vi "DSF.Engine.Framework.Create.Plugins.vi"(8 "error in (no error)":errorcluster, 10 "Plugin Configurations":refnum<class "DSF.Shared.Configuration.Plugin.lvclass">[](array[class]), 11 "Framework in":refnum<class "DSF.Engine.Framework.lvclass">) -> (0 "error out":errorcluster, 2 "Plugins":refnum<class "DSF.Engine.Plugin.lvclass">[](array[class]), 3 "Framework out":refnum<class "DSF.Engine.Framework.lvclass">)   [LabVIEW 2017, in "DSF.Engine.lvlib" / "DSF.Engine.Framework.lvclass"]
uses:
  DSF.Engine.Framework.lvclass
  Shared/Classes/Plugin/DSF.Shared.Configuration.Plugin.lvclass
  Plugin/DSF.Engine.Plugin.lvclass
  Plugins/UDP/DSF.Transceiver.UDP.lvclass
  C:/Git/DSF/Source/Engine/Classes/Transceiver/DSF.Engine.Transceiver.lvclass
  Shared/Classes/Plugin/DSF.Shared.Configuration.Plugin.lvclass/DSF.Shared.Configuration.Plugin.ctl
  DSF.Engine.Framework.lvclass/DSF.Engine.Framework.ctl
  Timing/DSF.Engine.Timing.lvclass
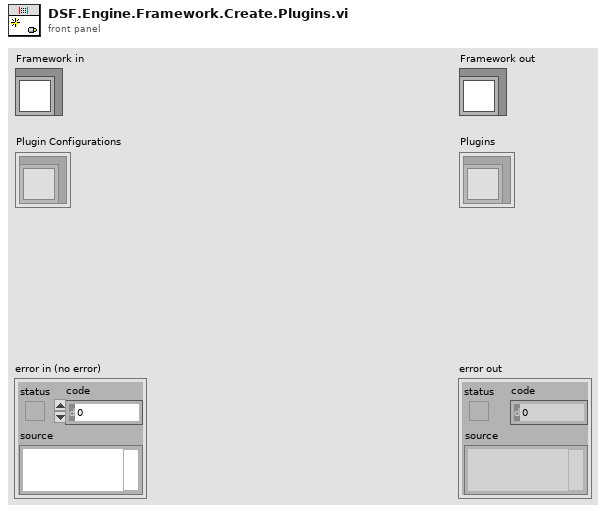
[diagram p1: front panel]
types:
  T1 = typedef "DSF.Shared.lvlib/DSF.Shared.Typedefs.Cycle Timing Factors.ctl" = cluster{"Priority":u64, "Decimation":u64, "Offset":u64}
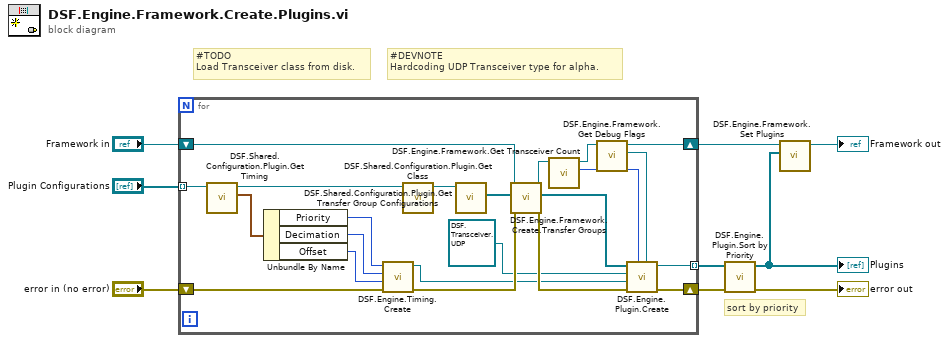
[diagram p0: block diagram]
diagram:
  # "#TODO\nLoad Transceiver class from disk."
  # "#DEVNOTE\nHardcoding UDP Transceiver type for alpha."
  # "sort by priority"
  n1 = for {
    shift-right: [w25] -> w7
    shift-left: "error in (no error)" -> [w26]
    shift-right: [w12] -> w3
    shift-left: "Framework in" -> [w21]
    tunnel: "Plugin Configurations" -> [w31] mode=indexing
    tunnel: [w17] -> w2 mode=indexing
    n2 = call "DSF.Shared.Configuration.Plugin.Get Timing.vi"("Plugin Configuration in"=w31) -> ("cycle timing"=w30:T1, "Plugin Configuration out"=w24:refnum<class "DSF.Shared.Configuration.Plugin.lvclass">)  [unwired: 9 in]
    n3 = Unbundle By Name(w30) -> ("Priority"=w27:u64, "Decimation"=w28:u64, "Offset"=w29:u64)
    n4 = call "DSF.Engine.Timing.Create.vi"("error in (no error)"=w26, "Offset"=w29, "Decimation"=w28, "Priority"=w27) -> ("error out"=w19:errorcluster, "Timing"=w16:refnum<class "DSF.Engine.Timing.lvclass">)  [unwired: 6 in]
    n5 = call "DSF.Shared.Configuration.Plugin.Get Class.vi"("Plugin Configuration in"=w24) -> ("Plugin Configuration out"=w23:refnum<class "DSF.Shared.Configuration.Plugin.lvclass">)  [unwired: 9 in, 1 out]
    n6 = call "DSF.Shared.Configuration.Plugin.Get Transfer Group Configurations.vi"("Plugin Configuration in"=w23) -> ("Transfer Group Configurations"=w22:refnum<class "DSF.Shared.Configuration.Transfer Group.lvclass">[])  [unwired: 9 in, 1 out]
    n7 = call "DSF.Engine.Framework.Create.Transfer Groups.vi"("error in (no error)"=w19, "Transfer Group Configurations"=w22, "Framework in"=w21) -> ("error out"=w18:errorcluster, "Transfer Groups"=w20:refnum<class "DSF.Engine.Transfer Group.lvclass">[], "Framework out"=w14:refnum<class "DSF.Engine.Framework.lvclass">)  [unwired: 6 in]
    n8 = call "DSF.Engine.Framework.Get Transceiver Count.vi"("Framework in"=w14) -> ("transceiver count"=w13:i32, "Framework out"=w11:refnum<class "DSF.Engine.Framework.lvclass">)  [unwired: 9 in]
    n9 = call "DSF.Engine.Framework.Get Debug Flags.vi"("Framework in"=w11) -> ("Debug Flags"=w10:refnum<class "DSF.Engine.Debug Flags.lvclass">, "Framework out"=w12:refnum<class "DSF.Engine.Framework.lvclass">)  [unwired: 9 in]
    n10 = call "DSF.Engine.Plugin.Create.vi"("Debug Flags"=w10, "transceiver count"=w13, "error in (no error)"=w18, "Timing"=w16, "Transceiver type"=refnum<class "DSF.Transceiver.UDP.lvclass"> refnum ("DSF UDP Transceiver"), "Transfer Groups"=w20) -> ("error out"=w25:errorcluster, "Plugin out"=w17:refnum<class "DSF.Engine.Plugin.lvclass">)  [unwired: 4 in]
  }
  n11 = call "DSF.Engine.Plugin.Sort by Priority.vi"("error in (no error)"=w7, "Plugins in"=w2) -> ("error out"=→"error out":errorcluster, "Plugins out"=w1:refnum<class "DSF.Engine.Plugin.lvclass">[])  [unwired: 8 in]
  "Plugins" <- w1
  n12 = call "DSF.Engine.Framework.Set Plugins.vi"("Plugins"=w1, "Framework in"=w3) -> ("Framework out"=→"Framework out":refnum<class "DSF.Engine.Framework.lvclass">)  [unwired: 9 in]
